vi "Configure Trigger.vi"(0 "VISA resource name":refnum<visa-resource-name>, 1 "Trigger Type (0:Untriggered)":u16(ring) items=["Untriggered", "Software Triggered", "Hardware Triggered"], 5 "Trigger Start Edge (0: Rising)":u16(ring) items=["Rising", "Falling"], 7 "Trigger Stop Edge (0: Rising)":u16(ring) items=["Rising", "Falling"], 9 "Trigger Stop Condition (1:Edge Triggering)":u16(ring)=1 items=["Number of Acquisitions", "Edge Triggering"], 11 "error in (no error)":errorcluster, 12 "Number of Acquisitions (100)":i32=100, 13 "Enable Continuous Trigger (Disabled)":bool) -> (4 "VISA resource name out":refnum<visa-resource-name>, 6 "Response":string[](array[string]), 15 "error out":errorcluster)   [LabVIEW 2024, in "Micron Optics sm130.lvlib"]
doc: "Configures the trigger settings such as trigger type, start and stop edge, stop conditions, number of acquisitions and enable continuous trigger."
uses:
  Micron Optics sm130.lvlib
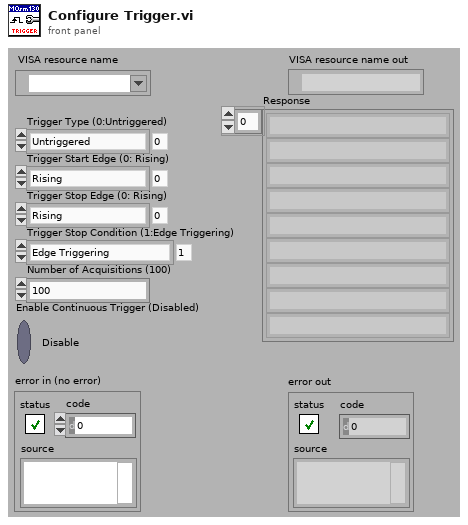
[diagram p1: front panel]
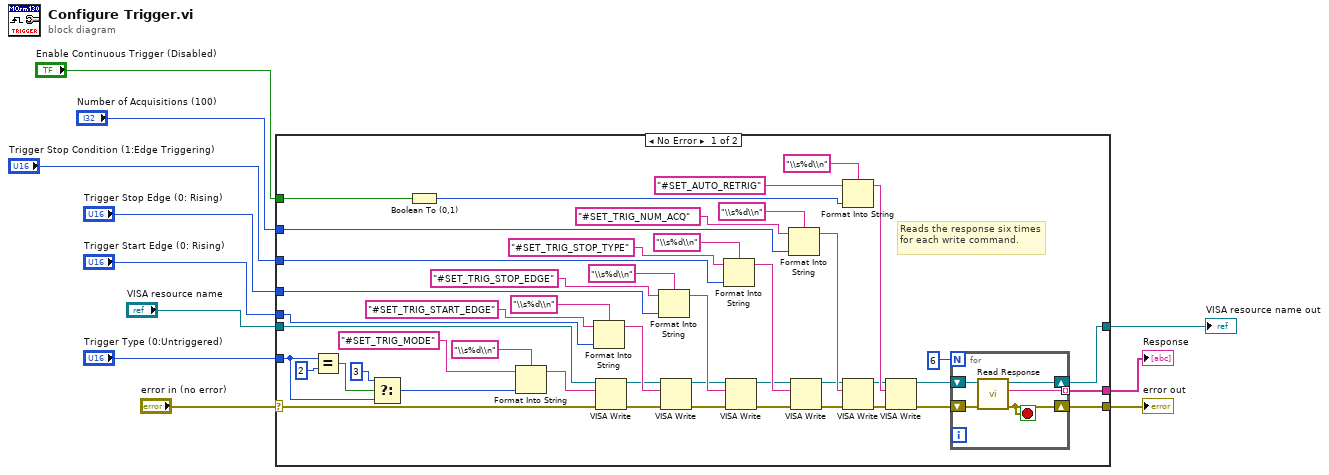
[diagram p0: block diagram]
diagram:
  n1 = case shown="No Error" "error in (no error)" {
    selector: "error in (no error)" -> [w12 w65]
    tunnel: "Trigger Start Edge (0: Rising)" -> [w54 _]
    tunnel: "Trigger Stop Edge (0: Rising)" -> [w50 _]
    tunnel: "Trigger Stop Condition (1:Edge Triggering)" -> [w47 _]
    tunnel: "Number of Acquisitions (100)" -> [w45 _]
    tunnel: "Enable Continuous Trigger (Disabled)" -> [w41 _]
    tunnel: "VISA resource name" -> [w21 w64]
    tunnel: [w20 w64] -> w5
    tunnel: [w19 w65] -> w4
    tunnel: [w18 _] -> w3
    tunnel: "Trigger Type (0:Untriggered)" -> [w14 _]
    frame No Error {
      # "Reads the response six times for each write command."
      n2 = Equal?(x=w14, y=u16 2) -> (x = y?=w16:bool)
      n3 = Select(t=u16 3, s=w16, f=w14) -> (s? t:f=w13:u16)
      n4 = Boolean To (0,1)(Boolean=w41) -> (0, 1=w40:i16)
      n5 = Format Into String(format string="\\s%d\\n", initial string="#SET_TRIG_MODE", w13) -> (resulting string=w56:string)  [unwired: 1 in, 1 out]
      n6 = Format Into String(format string="\\s%d\\n", initial string="#SET_TRIG_START_EDGE", w54) -> (resulting string=w39:string)  [unwired: 1 in, 1 out]
      n7 = VISA Write(VISA resource name=w21, write buffer=w56, error in (no error)=w12) -> (VISA resource name out=w23:refnum<visa-resource-name>, error out=w22:errorcluster)  [unwired: 1 out]
      n8 = Format Into String(format string="\\s%d\\n", initial string="#SET_TRIG_STOP_EDGE", w50) -> (resulting string=w38:string)  [unwired: 1 in, 1 out]
      n9 = VISA Write(VISA resource name=w23, write buffer=w39, error in (no error)=w22) -> (VISA resource name out=w25:refnum<visa-resource-name>, error out=w24:errorcluster)  [unwired: 1 out]
      n10 = Format Into String(format string="\\s%d\\n", initial string="#SET_TRIG_STOP_TYPE", w47) -> (resulting string=w37:string)  [unwired: 1 in, 1 out]
      n11 = VISA Write(VISA resource name=w25, write buffer=w38, error in (no error)=w24) -> (VISA resource name out=w26:refnum<visa-resource-name>, error out=w27:errorcluster)  [unwired: 1 out]
      n12 = Format Into String(format string="\\s%d\\n", initial string="#SET_TRIG_NUM_ACQ", w45) -> (resulting string=w36:string)  [unwired: 1 in, 1 out]
      n13 = VISA Write(VISA resource name=w26, write buffer=w37, error in (no error)=w27) -> (VISA resource name out=w29:refnum<visa-resource-name>, error out=w28:errorcluster)  [unwired: 1 out]
      n14 = Format Into String(format string="\\s%d\\n", initial string="#SET_AUTO_RETRIG", w40) -> (resulting string=w35:string)  [unwired: 1 in, 1 out]
      n15 = VISA Write(VISA resource name=w29, write buffer=w36, error in (no error)=w28) -> (VISA resource name out=w31:refnum<visa-resource-name>, error out=w30:errorcluster)  [unwired: 1 out]
      n16 = VISA Write(VISA resource name=w31, write buffer=w35, error in (no error)=w30) -> (VISA resource name out=w33:refnum<visa-resource-name>, error out=w32:errorcluster)  [unwired: 1 out]
      n17 = for {
        N: 6 -> [_]
        tunnel: [w60] -> w18 mode=indexing
        shift-right: [w59] -> w19
        shift-left: w32 -> [w62]
        shift-right: [w61] -> w20
        shift-left: w33 -> [w63]
        stop <- w59 stop-if-true
        n18 = call "Read Response.vi"("error in (no error)"=w62, "VISA resource name"=w63) -> ("error out"=w59:errorcluster, "Confirmation Response"=w60:string, "VISA resource name out"=w61:refnum<visa-resource-name>)  [unwired: 7 in]
      }
    }
    frame Error {
    }
  }
  "VISA resource name out" <- w5
  "error out" <- w4
  "Response" <- w3
